vi "0-Draw Boat Icon.vi"(4 "Position":cluster{"X":i32, "Y":i32}, 5 "Boat Bitmap":u32[][](array[numeric]), 7 "Image In":T1) -> (3 "Image Out":T1)   [LabVIEW 2011]
doc: "Draws the boat icon onto the map at the current location of the boat."
uses:
  <vilib>/vision/Image Controls.llb/IMAQ Image.ctl
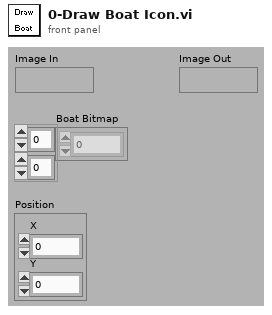
[diagram p1: front panel]
types:
  T1 = typedef "IMAQ Image.ctl" = refnum<image>
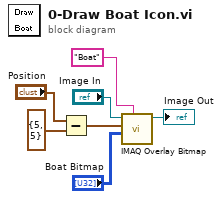
[diagram p0: block diagram]
diagram:
  n1 = Subtract(x="Position", y=cluster{"X":i32, "Y":i32} {"X"=5, "Y"=5}) -> (x-y=w7:cluster{"X":i32, "Y":i32})
  n2 = call "IMAQ Overlay Bitmap"("Group"="Boat", "Bitmap"="Boat Bitmap", "Top Left Point"=w7, "Image"="Image In") -> ("Image Out"=→"Image Out":T1)  [unwired: 1 in, 6 out]
